vi "Get area size.vi"(8 "error in (no error)":errorcluster, 10 "Sub Panel":refnum<vi>, 11 "DualScreenV in":refnum<class "DualScreenV.lvclass">) -> (0 "error out":errorcluster, 2 "Area size (px)":u32, 3 "DualScreenV out":refnum<class "DualScreenV.lvclass">)   [LabVIEW 2020, in "DualScreenV.lvlib" / "DualScreenV.lvclass"]
uses:
  DualScreenV.lvclass
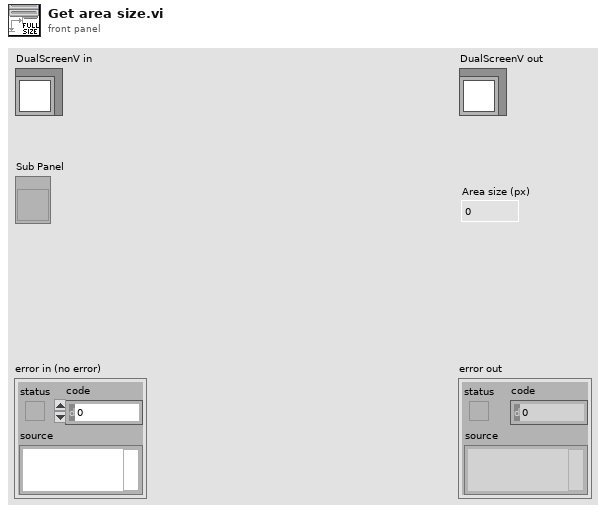
[diagram p1: front panel]
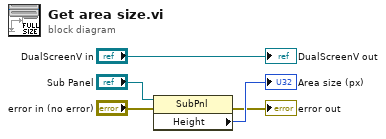
[diagram p0: block diagram]
diagram:
  n1 = property class="SubPnl"(reference="Sub Panel", error in="error in (no error)") -> (error out=→"error out":errorcluster, "Height"=→"Area size (px)":u32)  [unwired: 1 out]
  "DualScreenV out" <- "DualScreenV in"
